vi "GetAttributeViString.vi"(7 "AttributeValueBufferSize":i32=256, 8 "error in (no error)":errorcluster {"code" format="%.0x"}, 9 "AttributeID":u32(ring)=1150090 items=["ACP_DISPLAY_TEXT"=1150090, "CHANNELPOWER_DISPLAY_TITLE"=1190233, "DIGITAL_DEMOD_DISPLAY_TEXT"=1191586, "DIGITAL_DEMOD_SYNC_PATTERN"=1191655, "DIGITAL_DEMOD_TRACE_LIMIT_COMMENT"=1191671, "DIGITAL_DEMOD_TRACE_LIMIT_DESCRIPTION"=1191670, "DRIVER_SETUP"=1050007, "INSTRUMENT_FIRMWARE_REVISION"=1050510, "INSTRUMENT_MANUFACTURER"=1050511, "INSTRUMENT_MODEL"=1050512, "IO_RESOURCE_DESCRIPTOR"=1050304, "LOGICAL_NAME"=1050305, "MONITOR_DISPLAY_TITLE"=1190351, "OCCUPIED_BANDWIDTH_DISPLAY_TEXT"=1190390, "POWER_STATISTICS_DISPLAY_TEXT"=1190433, "SEMASK_DISPLAY_TEXT"=1190491, "SPECIFIC_DRIVER_DESCRIPTION"=1050514, "SPECIFIC_DRIVER_PREFIX "=1050302, "SPECIFIC_DRIVER_REVISION"=1050551, "SPECIFIC_DRIVER_VENDOR"=1050513, "SPURIOUS_EMISSIONS_DISPLAY_TEXT"=1190519, "SUPPORTED_INSTRUMENT_MODELS"=1050327, "SYSTEM_SERIAL_NUMBER"=1191769, "WAVEFORM_DISPLAY_TITLE"=1190543], 10 "RepCapIdentifier":string, 11 "instrument handle":refnum<k15>) -> (0 "error out":errorcluster {"code" format="%.0x"}, 2 "AttributeValue":string, 3 "instrument handle out":refnum<k15>)   [LabVIEW 2021, in "Keysight XSAnVMA.lvlib"]
doc: "Gets a String attribute from the instrument driver.\nThe following Attributes are supported:\nACP_DISPLAY_TEXT\nCHANNELPOWER_DISPLAY_TITLE\nDIGITAL_DEMOD_DISPLAY_TEXT\nDIGITAL_DEMOD_SYNC_PATTERN\nDIGITAL_DEMOD_TRACE_LIMIT_COMMENT\nDIGITAL_DEMOD_TRACE_LIMIT_DESCRIPTION\nDRIVER_SETUP\nINSTRUMENT_FIRMWARE_REVISION\nINSTRUMENT_MANUFACTURER\nINSTRUMENT_MODEL\nIO_RESOURCE_DESCRIPTOR\nLOGICAL_NAME\nMONITOR_DISPLAY_TITLE\nOCCUPIED_BANDWIDTH_DISPLAY_TEXT\nPOWER_STATISTICS_DISPLAY_TEXT\nSEMASK_DISPLAY_TEXT\nSPECIFIC_DRIVER_DESCRIPTION\nSPECIFIC_DRIVER_REVISION\nSPECIFIC_DRIVER_PREFIX\nSPECIFIC_DRIVER_VENDOR\nSPURIOUS_EMISSIONS_DISPLAY_TEXT\nSUPPORTED_INSTRUMENT_MODELS\nSYSTEM_SERIAL_NUMBER\nWAVEFORM_DISPLAY_TITLE"
uses:
  <instrlib>/Keysight XSAnVMA/Keysight XSAnVMA.lvlib
  KtXSAnVMA_64.dll
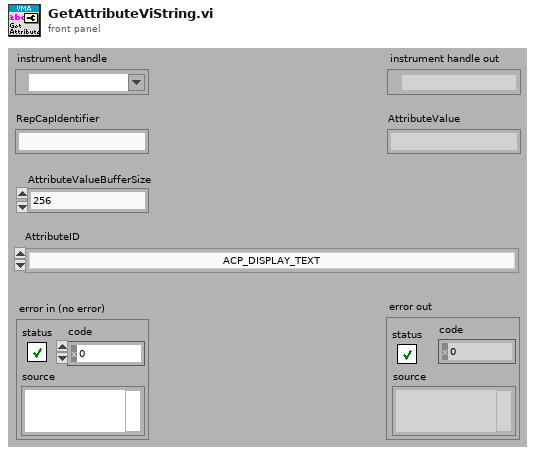
[diagram p1: front panel]
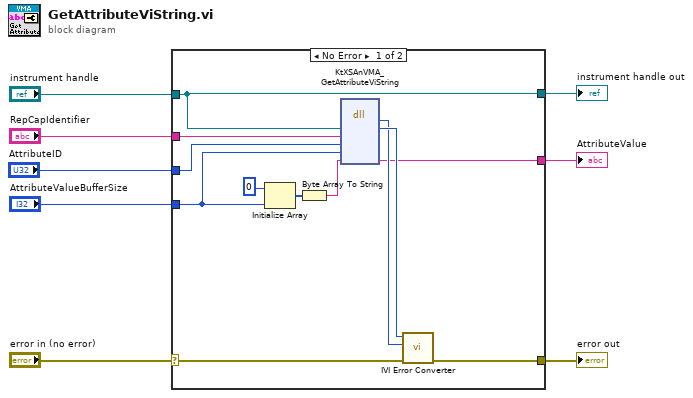
[diagram p0: block diagram]
diagram:
  n1 = case shown="No Error" "error in (no error)" {
    selector: "error in (no error)" -> [w18 w22]
    tunnel: [w17 w22] -> w8
    tunnel: "instrument handle" -> [w10 w21]
    tunnel: "RepCapIdentifier" -> [w16 _]
    tunnel: "AttributeID" -> [w15 _]
    tunnel: "AttributeValueBufferSize" -> [w9 _]
    tunnel: [w11 _] -> w3
    tunnel: [w10 w21] -> w2
    frame No Error {
      n2 = Initialize Array(u8 0 ("element"), w9) -> (w13:u8[])
      n3 = Byte Array To String(unsigned byte array=w13) -> (string=w14:string)
      n4 = dll-call lib="KtXSAnVMA**.dll" fn="KtXSAnVMA_GetAttributeViString"("Vi"=w10, "RepCapIdentifier"=w16, "AttributeID"=w15, "AttributeValueBufferSize"=w9, "AttributeValue"=w14) -> ("return type"=w19:i32, "Vi"=w20:u32, "AttributeValue"=w11:string)  [unwired: 6 in, 2 out]
      n5 = call <instrlib>:"IVI Error Converter.vi"("error in (no error)"=w18, "IVI error code (0)"=w19, "instrument handle"=w20) -> ("error out"=w17:errorcluster)  [unwired: 7 in, 1 out]
    }
    frame Error {
    }
  }
  "error out" <- w8
  "instrument handle out" <- w2
  "AttributeValue" <- w3
